vi "Output_Counter_ENSW.vi"() -> ()   [LabVIEW 2018]
uses:
  <vilib>/DAQmx/create/channels.llb/DAQmx Create Channel (CO-Pulse Generation-Frequency).vi
  <vilib>/DAQmx/configure/timing.llb/DAQmx Timing (Implicit).vi
panel:
  in  "정지":bool
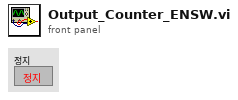
[diagram p1: front panel]
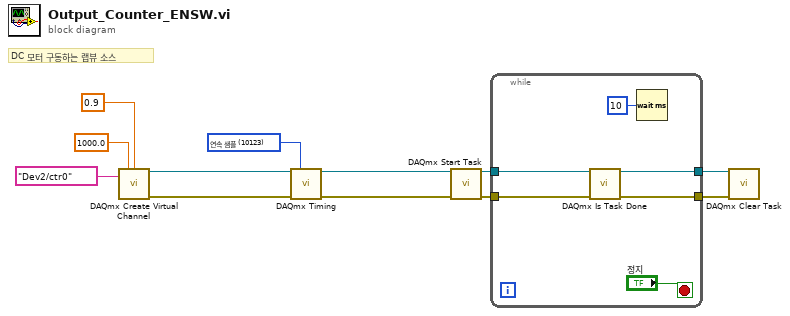
[diagram p0: block diagram]
diagram:
  w1 = 10123 items=["유한 샘플"=10178, "연속 샘플"=10123, "하드웨어 타이밍에 의한 단일 포인트"=12522] ("sample mode")
  # "DC 모터 구동하는 랩뷰 소스"
  n1 = call-poly <vilib>:"DAQmx Create Virtual Channel.vi"("frequency"=1000.0, "duty cycle"=0.9, "counter"=tag "Dev2/ctr0") -> ("task out"=w12:refnum<k21>, "error out"=w11:errorcluster)  [unwired: 11 in]
  n2 = call-poly <vilib>:"DAQmx Timing.vi"("task/channels in"=w12, "sample mode"=w1, "error in"=w11) -> ("task out"=w10:refnum<k21>, "error out"=w9:errorcluster)  [unwired: 11 in]
  n3 = call <vilib>:"DAQmx Start Task.vi"("task/channels in"=w10, "error in"=w9) -> ("task out"=w8:refnum<k21>, "error out"=w7:errorcluster)  [unwired: 12 in]
  n4 = while {
    tunnel: w8 -> [w18]
    tunnel: w7 -> [w17]
    tunnel: [w16] -> w6
    tunnel: [w15] -> w5
    stop <- "정지" stop-if-true
    n5 = call <vilib>:"DAQmx Is Task Done.vi"("task/channels in"=w18, "error in"=w17) -> ("task out"=w16:refnum<k21>, "error out"=w15:errorcluster)  [unwired: 11 in, 1 out]
    n6 = Wait (ms)(milliseconds to wait=u32 10 ("대기 시간 (ms)")) -> ()  [unwired: 1 out]
  }
  n7 = call <vilib>:"DAQmx Clear Task.vi"("task in"=w6, "error in"=w5) -> ()  [unwired: 13 in, 1 out]
